vi "Sync.vi"(8 "error in (no error)":errorcluster, 10 "file ref":refnum<file>, 11 "rollover trigger in":refnum<class "RolloverTrigger.lvclass">) -> (0 "error out":errorcluster, 3 "rollover trigger out":refnum<class "RolloverTrigger.lvclass">)   [LabVIEW 2018, in "GLog.lvlib" / "RolloverTrigger.lvclass"]
doc: "Synchronizes the rollover trigger with the new file."
uses:
  RolloverTrigger.lvclass
panel:
  # "Connector Pane"
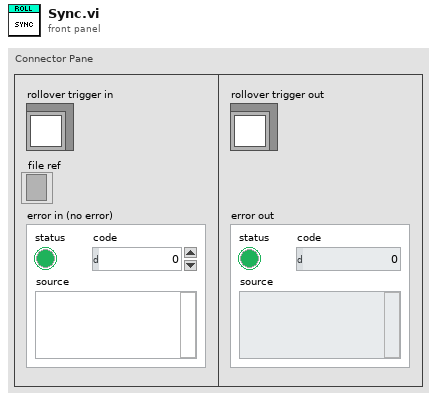
[diagram p1: front panel]
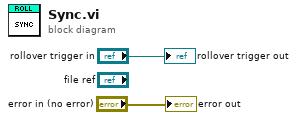
[diagram p0: block diagram]
diagram:
  "rollover trigger out" <- "rollover trigger in"
  "error out" <- "error in (no error)"
